vi "Overview Init.vi"(3 "Container State":T3, 4 "Previous State":variant, 5 "Previous Version":T2) -> (2 "Current State":T1={"Numeric"=0.0, "Fill Plots"=FALSE, "Cursor Redraw"=TRUE, "XYGraph Refnum"=refnum})   [LabVIEW 2020, in "Overview XControl.xctl"]
uses:
  Overview XControl.xctl
  Overview State.ctl
  <vilib>/_xctls/Container State.ctl
  <vilib>/_xctls/Version.ctl
  <vilib>/_xctls/XControlSupport.lvlib
panel:
  in  "Default Indicator State":T1={"Numeric"=0.0, "Fill Plots"=FALSE, "Cursor Redraw"=TRUE, "XYGraph Refnum"=refnum}
  in  "Default Control State":T1={"Numeric"=0.0, "Fill Plots"=FALSE, "Cursor Redraw"=TRUE, "XYGraph Refnum"=refnum}
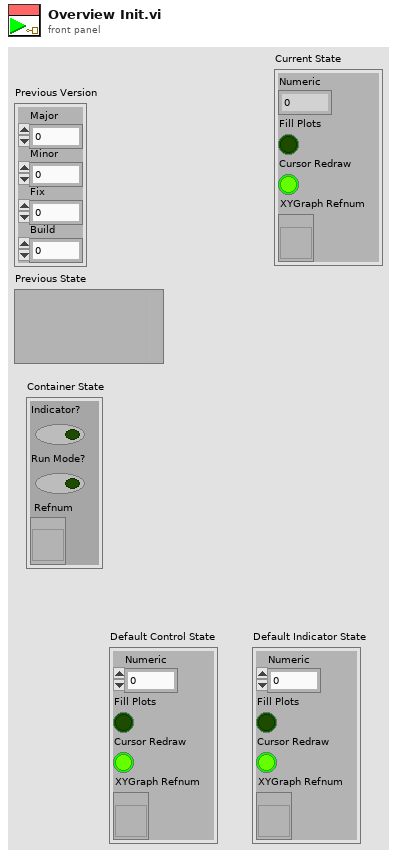
[diagram p1: front panel]
types:
  T1 = typedef "Overview XControl.xctl/Overview State.ctl" = cluster{"Numeric":dbl, "Fill Plots":bool, "Cursor Redraw":bool, "XYGraph Refnum":refnum<vi>}
  T2 = typedef "XControlSupport.lvlib/Version.ctl" = cluster{"Major":u16, "Minor":u16, "Fix":u16, "Build":u16}
  T3 = typedef "XControlSupport.lvlib/Container State.ctl" = cluster{"Indicator?":bool, "Run Mode?":bool, " Refnum":refnum<vi>}
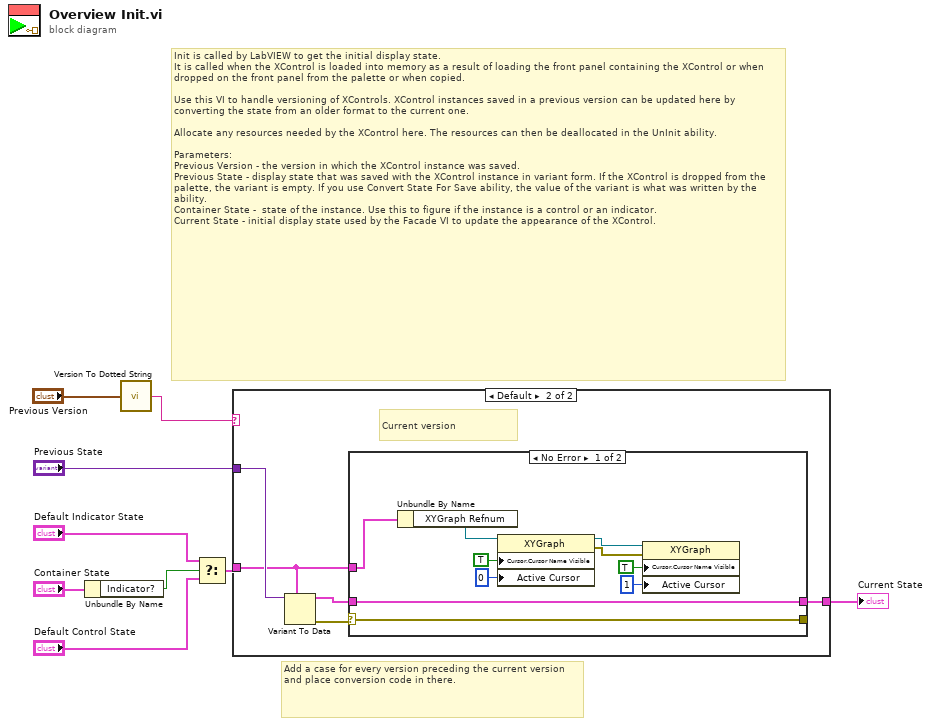
[diagram p0: block diagram]
diagram:
  # "Add a case for every version preceding the current version and place conversion code in there."
  # "Init is called by LabVIEW to get the initial display state.\nIt is called when the XControl is loaded into memory as a result of loading the front panel containing the XControl or when dropped on the front panel from the palette or when copied.\n\nUse this VI to handle versioning of XControls. XControl instances saved in a previous version can be updated here by converting the state from an older format to the current one.\n\nAllocate any resources needed by the XControl here. The resources can then be deallocated in the UnInit ability.\n\nParameters:\nPrevious Version - the version in which the XControl instance was saved.\nPrevious State - display state that was saved with the XControl instance in variant form. If the XControl is dropped from the palette, the variant is empty. If you use Convert State For Save ability, the value of the variant is what was written by the ability. \nContainer State -  state of the instance. Use this to figure if the instance is a control or an indicator.\nCurrent State - initial display state used by the Facade VI to update the appearance of the XControl."
  n1 = Unbundle By Name("Container State") -> ("Indicator?"=w4:bool)
  n2 = call <vilib>:"Version To Dotted String.vi"("Version"="Previous Version") -> ("String Version"=w1:string)
  n3 = Select(t="Default Indicator State", s=w4, f="Default Control State") -> (s? t:f=w3:T1)
  n4 = case shown="Default" w1 {
    tunnel: "Previous State" -> [_ w15]
    tunnel: [w10 w11] -> w8
    tunnel: w3 -> [w10 w12]
    frame "0.0.0.0" {
      # "Just created, use default state"
    }
    frame Default {
      # "Current version"
      n5 = Variant To Data(type=w12, Variant=w15) -> (data=w13:T1, error out=w14:errorcluster)  [unwired: 1 in]
      n6 = case shown="No Error" w14 {
        selector: w14 -> [w25 w26]
        tunnel: w13 -> [w24 _]
        tunnel: [w24 w27] -> w11
        tunnel: w12 -> [w23 w27]
        tunnel: [w25 w26] -> _
        frame No Error {
          n7 = Unbundle By Name(w23) -> ("XYGraph Refnum"=w22:refnum<vi>)
          n8 = property class="XYGraph"(reference=w22, "Cursor.Cursor Name Visible"=TRUE, "Active Cursor"=u32 0) -> (reference out=w17:refnum<vi>, error out=w16:errorcluster)  [unwired: 1 in]
          n9 = property class="XYGraph"(reference=w17, error in=w16, "Cursor.Cursor Name Visible"=TRUE, "Active Cursor"=u32 1) -> ()  [unwired: 2 out]
        }
        frame Error {
          # "Error converting previously \nsaved state. Use default instead."
        }
      }
    }
  }
  "Current State" <- w8
